vi "Cast To Variant (Object).vi"(8 "error in (no error)":errorcluster, 9 "datatype and defaults":variant, 11 "JSON Value in":refnum<class "JSON Value.lvclass">) -> (0 "error out":errorcluster, 2 "Variant":variant)   [LabVIEW 2016, in "JSFL Variant Support.lvlib"]
doc: "Populates a variant with the data contained in the given JSON instance. Valid types for datatype and defaults are: string, boolean, double, and a cluster of named controls of strings, booleans, doubles, or nested clusters.\n\nIf a given cluster contains values that aren't present in the JSON Object instance, the value in the datatype and defaults control is used instead and the defaulted keys output will contain the name of the path in the cluster to the control."
uses:
  JSFL Variant Support.lvlib
  JSON Value.lvclass
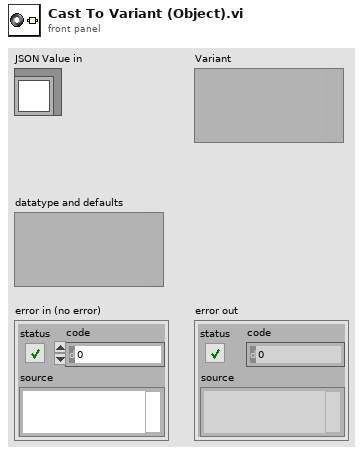
[diagram p1: front panel]
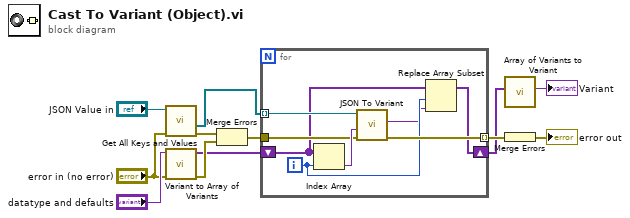
[diagram p0: block diagram]
diagram:
  n1 = call "Get All Keys and Values.vi"("error in"="error in (no error)", "JSON Value in"="JSON Value in") -> ("error out"=w6:errorcluster, "values"=w3:refnum<class "JSON Value.lvclass">[])  [unwired: 7 in, 1 out]
  n2 = call "Variant to Array of Variants.vi"("error in (no error)"="error in (no error)", "variant"="datatype and defaults") -> ("error out"=w5:errorcluster, "Array"=w2:variant[])  [unwired: 8 in]
  n3 = Merge Errors(w6, w5) -> (w4:errorcluster)
  n4 = for {
    tunnel: [w20] -> w11 mode=indexing
    tunnel: w3 -> [w19] mode=indexing
    tunnel: w4 -> [w17]
    shift-right: [w13] -> w1
    shift-left: w2 -> [w16]
    i -> [w15]
    n5 = Index Array(array=w16, index=w15) -> (element=w18:variant)
    n6 = call "JSON To Variant.vi"("error in (no error)"=w17, "datatype and defaults"=w18, "JSON Value in"=w19) -> ("error out"=w20:errorcluster, "Variant"=w14:variant)  [unwired: 7 in]
    n7 = Replace Array Subset(array=w16, new element=w14, index=w15) -> (w13:variant[])
  }
  n8 = call "Array of Variants to Variant.vi"("Array"=w1) -> ("Variant"=→"Variant":variant)  [unwired: 10 in]
  n9 = Merge Errors(w11) -> (→"error out":errorcluster)
